vi "Global allarmi procedure.vi"() -> ()   [LabVIEW 2019]
panel:
  out "Allarme Presente":bool
  out "carico resistivo non trovato":bool
  out "Allarme Apri potenza":bool
  out "Allarme Start Alimentatore":bool
  out "Allarme Start inverter":bool
  out "Allarme Start potenza":bool
  out "Allarme Abilita potenza":bool
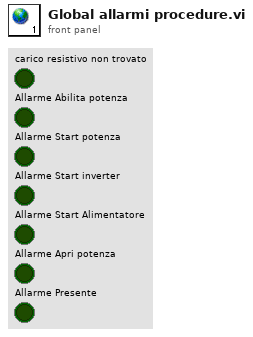
[diagram p1: front panel]
diagram:
